vi "Test Transcriptor LabVIEW to C code 1.vi"() -> ()   [LabVIEW 2014]
panel:
  out "Transcripted code":string
  out "error out":errorcluster
  in  "vi path":path=path "C:/Users/lubo/Documents/LabView/LabVIEW-Universal-Transcriptor/Test/Examples For Parsing/Blink 2.vi"
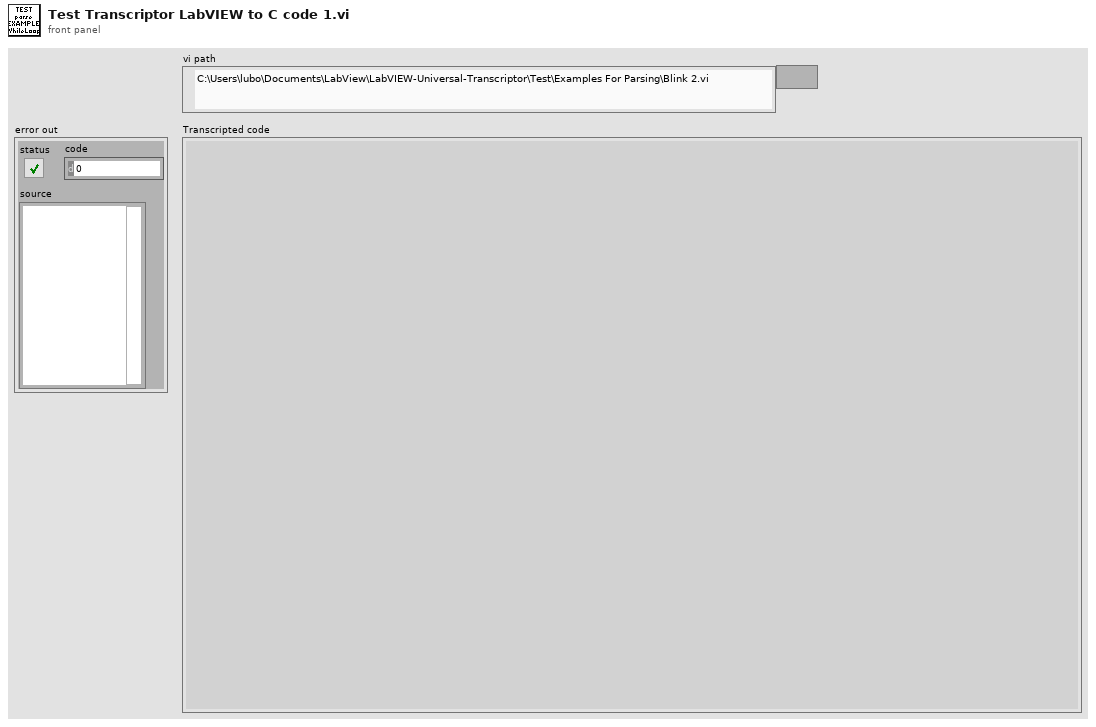
[diagram p1: front panel]
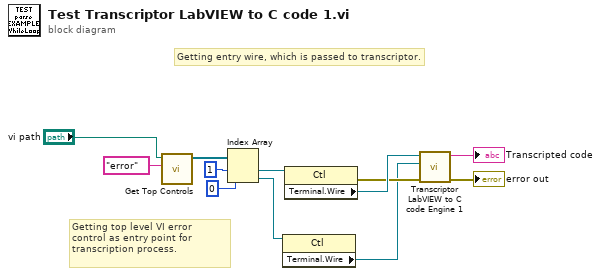
[diagram p0: block diagram]
diagram:
  # "Getting entry wire, which is passed to transcriptor."
  # "Getting top level VI error control as entry point for transcription process."
  n1 = call "Get Top Controls.vi"("DataType"="error", "vi path"="vi path") -> ("Controls Referencies Array"=w10:refnum<vi>[])  [unwired: 8 in, 1 out]
  n2 = Index Array(array=w10, index #1=1 ("index"), index #2=0 ("index")) -> (element #1=w9:refnum<vi>, element #2=w3:refnum<vi>)
  n3 = property on="Property Node" class="Ctl"(reference=w3) -> ("Terminal.Wire"=w2:refnum<vi>)  [unwired: 1 in, 2 out]
  n4 = property on="Property Node" class="Ctl"(reference=w9) -> (error out=w6:errorcluster, "Terminal.Wire"=w8:refnum<vi>)  [unwired: 1 in, 1 out]
  n5 = call "Transcriptor LabVIEW to C code Engine 1.vi"("error in (no error)"=w6, "GObject stop"=w2, "GObject start"=w8) -> ("error out"=→"error out":errorcluster, "Transcripted code"=→"Transcripted code":string)  [unwired: 7 in]
